vi "Data Check.vi"(0 "RFFE Reg0Write Command in":refnum<class "RFFE Reg0Write Command.lvclass">, 11 "error in (no error)":errorcluster) -> (4 "RFFE Reg0Write Command out":refnum<class "RFFE Reg0Write Command.lvclass">, 15 "error out":errorcluster)   [LabVIEW 2018, in "MIPI RFFE API.lvlib" / "RFFE Reg0Write Command.lvclass"]
uses:
  RFFE Reg0Write Command.lvclass
  Register Data.ctl
  RFFE Reg0Write Command.lvclass/RFFE Reg0Write Command.ctl
  Command/RFFE Command.lvclass
  MIPI RFFE API.lvlib
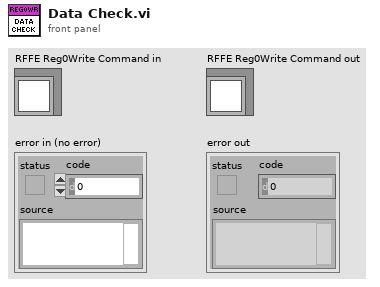
[diagram p1: front panel]
types:
  T1 = typedef "MIPI RFFE API.lvlib/Register Data.ctl" = u8
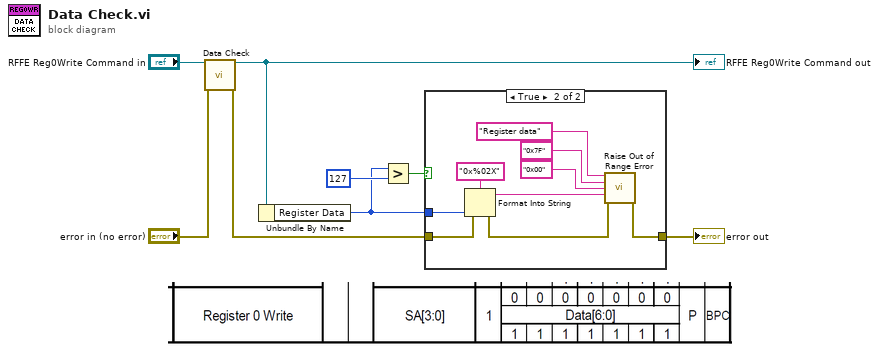
[diagram p0: block diagram]
diagram:
  n1 = call-parent "Data Check.vi"("RFFE Command in"="RFFE Reg0Write Command in", "error in (no error)"="error in (no error)") -> ("RFFE Command out"=w6:refnum<class "RFFE Reg0Write Command.lvclass">, "error out"=w5:errorcluster)  [unwired: 12 in]
  "RFFE Reg0Write Command out" <- w6
  n2 = Unbundle By Name(w6) -> ("Register Data"=w1:T1)
  n3 = Greater?(x=w1, y=T1 127) -> (0:w2:bool)
  n4 = case shown="True" w2 {
    tunnel: w5 -> [w9 w10]
    tunnel: [w9 w18] -> w4
    tunnel: w1 -> [_ w13]
    frame False {
    }
    frame True {
      n5 = Format Into String(format string="0x%02X", error in=w10, w13) -> (resulting string=w12:string, error out=w11:errorcluster)  [unwired: 1 in]
      n6 = call "Raise Out of Range Error.vi"("Parameter Name"="Register data", "Upper Limit"="0x7F" ("Lower Limit"), "Lower Limit"="0x00" ("Upper Limit"), "As Found"=w12, "error in (no error)"=w11) -> ("error out"=w18:errorcluster)  [unwired: 10 in]
    }
  }
  "error out" <- w4
